vi "Internal Error Control Indices Map.vi"(7 "Set":bool, 11 "Error Out Indices Map in":map{refnum<vi>, i32}(c390)) -> (3 "Error Out Indices Map out":map{refnum<vi>, i32}(c390))   [LabVIEW 2025, in "I2C Bus Monitor UI.lvlib"]
uses:
  I2C Bus Monitor UI.lvlib
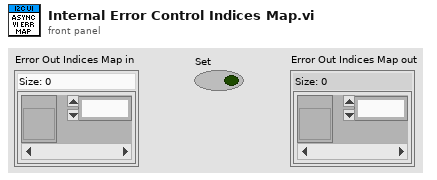
[diagram p1: front panel]
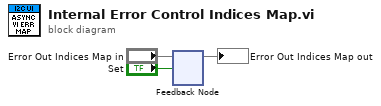
[diagram p0: block diagram]
diagram:
  n1 = feedback-in #1("Error Out Indices Map in", "Set") -> ()
  n2 = feedback #1() -> (→"Error Out Indices Map out":map{refnum<vi>, i32})  [unwired: 1 in]
